vi "update_nested_actors_attributes.vi"(8 "error in (no error)":errorcluster, 11 "root_actor in":refnum<class "root_actor.lvclass">) -> (0 "error out":errorcluster, 3 "root_actor out":refnum<class "root_actor.lvclass">)   [LabVIEW 2025, in "root_actor.lvlib" / "root_actor.lvclass"]
uses:
  root_actor.lvclass
  root_actor.lvclass/root_actor.ctl
  UDP_receiver/UDP_receiver Messages/update_attributes Msg/update_attributes Msg.lvclass/update_attributes Msg.ctl
  <vilib>/ActorFramework/Message Enqueuer/Message Enqueuer.lvclass/Message Enqueuer.ctl
  UDP_transmitter/UDP_transmitter Messages/update_attributes Msg/update_attributes Msg.lvclass/update_attributes Msg.ctl
  <vilib>/ActorFramework/Message Enqueuer/Enqueue.vi
  UDP_receiver/UDP_receiver Messages/update_attributes Msg/update_attributes Msg.lvclass
  Applications/National Instruments/LabVIEW 2025 64-bit/vi.lib/ActorFramework/Message/Message.lvclass
  UDP_transmitter/UDP_transmitter Messages/update_attributes Msg/update_attributes Msg.lvclass
  <vilib>/ActorFramework/Message Priority Queue/Priority Enqueue.vi
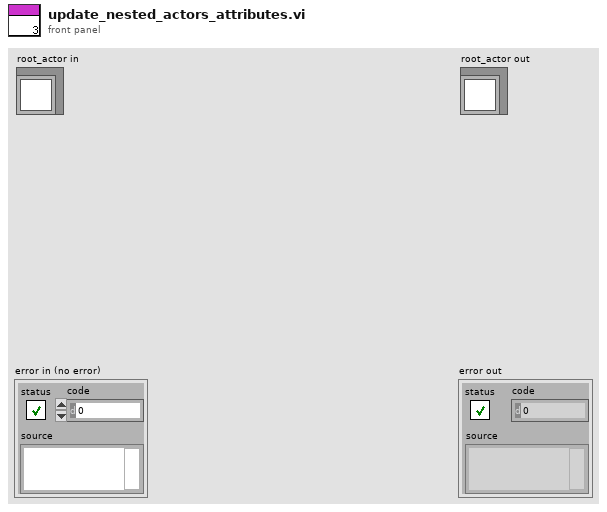
[diagram p1: front panel]
types:
  T1 = map{string, refnum<class "Message Enqueuer.lvclass">}
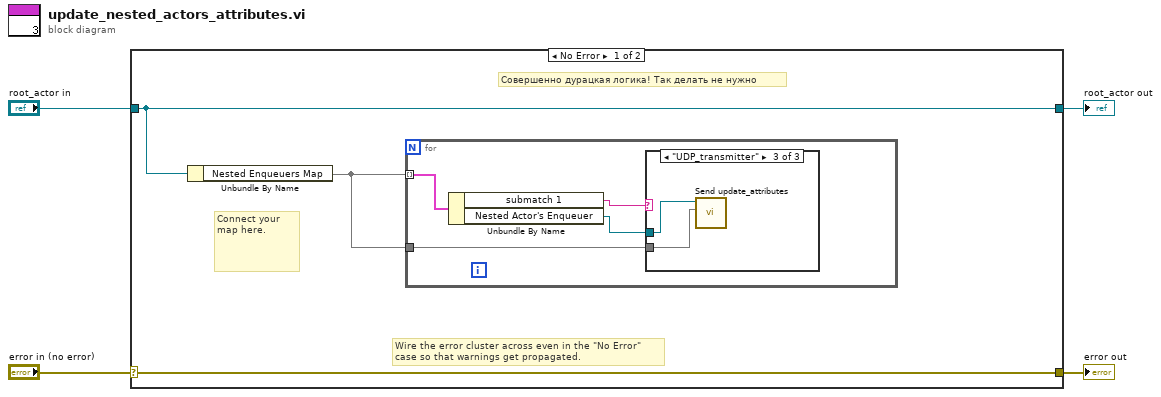
[diagram p0: block diagram]
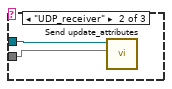
[diagram p3: hidden frame]
diagram:
  n1 = case shown="No Error" "error in (no error)" {
    selector: "error in (no error)" -> [w7 w17]
    tunnel: [w7 w17] -> w3
    tunnel: [w6 w16] -> w1
    tunnel: "root_actor in" -> [w6 w16]
    frame No Error {
      # "Совершенно дурацкая логика! Так делать не нужно"
      # "Connect your map here."
      # "Wire the error cluster across even in the \"No Error\"\ncase so that warnings get propagated."
      n2 = Unbundle By Name(w6) -> ("Nested Enqueuers Map"=w5:T1)
      n3 = for {
        tunnel: w5 -> [w11] mode=indexing
        tunnel: w5 -> [w8]
        n4 = Unbundle By Name(w11) -> ("submatch 1"=w10:string, "Nested Actor's Enqueuer"=w9:refnum<class "Message Enqueuer.lvclass">)
        n5 = case shown="\"UDP_transmitter\"" w10 {
          tunnel: w9 -> [_ w13 w15]
          tunnel: w8 -> [_ w12 w14]
          frame "False", Default {
          }
          frame "UDP_receiver" {
            n6 = call "Send update_attributes.vi"("Nested Enqueuers Map"=w12, "Message Enqueuer"=w13) -> ()  [unwired: 8 in, 2 out]
          }
          frame "UDP_transmitter" {
            n7 = call "Send update_attributes.vi"("Nested Enqueuers Map"=w14, "Message Enqueuer"=w15) -> ()  [unwired: 8 in, 2 out]
          }
        }
      }
    }
    frame Error {
    }
  }
  "error out" <- w3
  "root_actor out" <- w1
